vi "Subvi timeout.vi"(8 "Timeout_tick":i16, 10 "Input":bool) -> (2 "Timeout":bool)   [LabVIEW 2017]
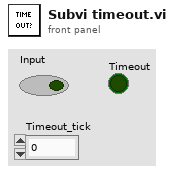
[diagram p1: front panel]
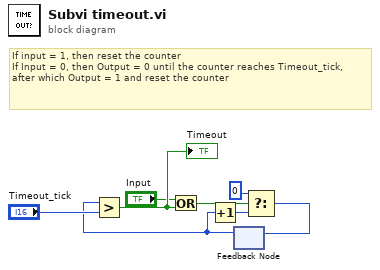
[diagram p0: block diagram]
diagram:
  # "If input = 1, then reset the counter\nIf Input = 0, then Output = 0 until the counter reaches Timeout_tick,\nafter which Output = 1 and reset the counter"
  n1 = feedback #1() -> (w1:i16)  [unwired: 1 in]
  n2 = Greater?(x=w1, y="Timeout_tick") -> (0:w5:bool)
  "Timeout" <- w5
  n3 = Or(x="Input", y=w5) -> (x .or. y?=w8:bool)
  n4 = Increment(x=w1) -> (x+1=w3:i16)
  n5 = Select(t=i16 0, s=w8, f=w3) -> (s? t:f=w2:i16)
  n6 = feedback-in #1(w2) -> ()
